vi "Connect.vi"(8 "error in (no error)":errorcluster, 11 "ByteGSWebAPI_New in":refnum<class "ByteGSWebAPI_New.lvclass">) -> (0 "error out":errorcluster, 3 "ByteGSWebAPI_New out":refnum<class "ByteGSWebAPI_New.lvclass">)   [LabVIEW 2019, in "ByteGSWebAPI.lvlib" / "ByteGSWebAPI_New.lvclass"]
doc: "Effettua la connessione al server e richiede il token di accesso.\nIn caso in cui la connessione non avvenga o il token non venga restituito (password o user errati), restituisce un errore."
uses:
  ByteGSWebAPI_New.lvclass
  <vilib>/Bytelabs/BIC-ByteIniConfig/ByteIniConfig.lvlib
  <vilib>/httpClient/LabVIEWHTTPClient.lvlib
  <vilib>/Bytelabs/BIC-ByteIniConfig/Read/ReadString.vi
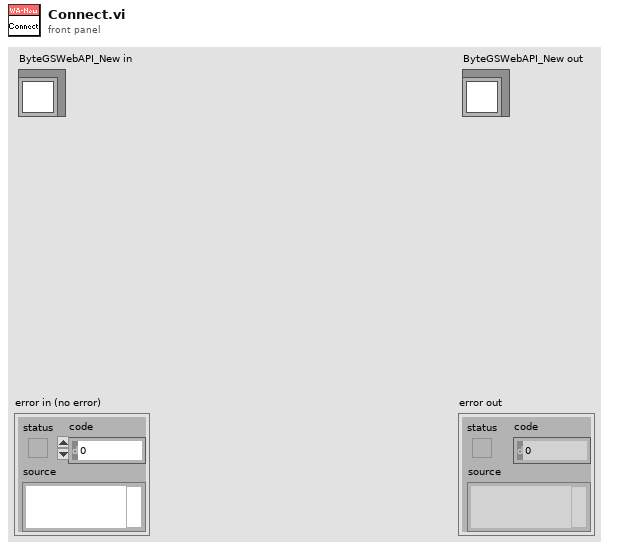
[diagram p1: front panel]
types:
  T1 = typedef "LabVIEWHTTPClient.lvlib/ClientHandle.ctl" = refnum<k1>
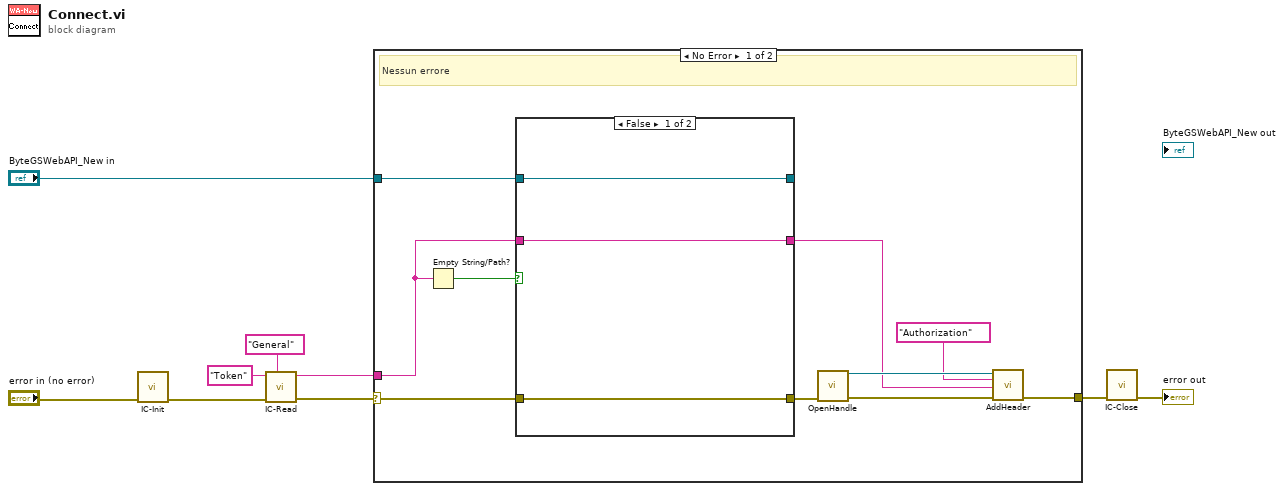
[diagram p0: block diagram]
diagram:
  n1 = call <vilib>:"IC-Init.vi"("error in (no error)"="error in (no error)") -> ("error out"=w8:errorcluster)  [unwired: 10 in]
  n2 = call-poly <vilib>:"IC-Read.vi"("section"="General", "error in (no error)"=w8, "key"="Token") -> ("error out"=w5:errorcluster, "String"=w4:string)  [unwired: 7 in]
  n3 = case shown="No Error" w5 {
    selector: w5 -> [w17 _]
    tunnel: w4 -> [w12 _]
    tunnel: "ByteGSWebAPI_New in" -> [w18 _]
    tunnel: [w10 _] -> w1
    frame No Error {
      # "Nessun errore"
      n4 = Empty String/Path?(string/path=w12) -> (empty?=w19:bool)
      n5 = case shown="False" w19 {
        tunnel: w18 -> [w20 w23]
        tunnel: w17 -> [w22 w24]
        tunnel: [w22 w24] -> w16
        tunnel: w12 -> [w21 _]
        tunnel: [w21 _] -> w11
        tunnel: [w20 w23] -> _
        frame False {
        }
        frame True {
          # "Qui sarà implementata \nla UI per l'inserimento del token"
        }
      }
      n6 = call <vilib>:"OpenHandle.vi"("error in (no error)"=w16) -> ("client handle out"=w14:T1, "error out"=w15:errorcluster)  [unwired: 13 in]
      n7 = call <vilib>:"AddHeader.vi"("client handle"=w14, "header"="Authorization", "value"=w11, "error in (no error)"=w15) -> ("error out"=w10:errorcluster)  [unwired: 10 in, 1 out]
    }
    frame Error {
      # "Errore dovuto al file setting"
    }
  }
  n8 = call <vilib>:"IC-Close.vi"("error in (no error)"=w1) -> ("error out"=→"error out":errorcluster)  [unwired: 10 in]
